vi "Register File Sink as Default.vi"(8 "error in (no error)":errorcluster, 11 "Path":path) -> (0 "error out":errorcluster)   [LabVIEW 2020, in "LV Log.lvlib"]
uses:
  LV Log.lvlib
  Sinks/File Sink/File Sink.lvclass
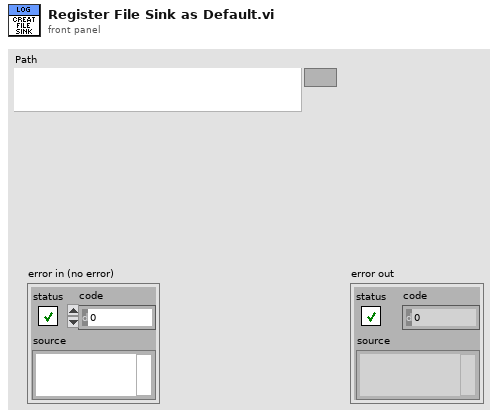
[diagram p1: front panel]
types:
  T1 = enum16{"Init", "Get Logger", "Register Sink", "Set Global Debug Level", "Get Sinks"}
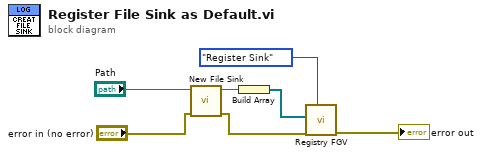
[diagram p0: block diagram]
diagram:
  n1 = call "New File Sink.vi"("error in (no error)"="error in (no error)", "File Path"="Path") -> ("error out"=w3:errorcluster, "File Sink out"=w5:refnum<class "File Sink.lvclass">)  [unwired: 8 in]
  n2 = Build Array(w5) -> (w1:refnum<class "File Sink.lvclass">[])
  n3 = call "Registry FGV.vi"("State (Get Logger)"=T1."Register Sink", "error in (no error)"=w3, "Sink(s)"=w1) -> ("error out"=→"error out":errorcluster)  [unwired: 5 in, 3 out]
